vi "FPGAmain_5782_PIDtest.vi"() -> ()   [LabVIEW 2013]
uses:
  FPGA/DataMode.ctl
  FPGA/Input_5782/5782_states.ctl
  <vilib>/Platform/TimedLoop/XDataNode/timing_clust.ctl
  <vilib>/Platform/TimedLoop/XDataNode/nitl_modes.ctl
  <vilib>/Platform/TimedLoop/XDataNode/wakeup.ctl
  <vilib>/rvi/Emulation/niFpgaSctlEmulationGetInTimedLoop.vi
  <vilib>/rvi/Emulation/niFpgaEmulationReportErrorSimple.vi
  <vilib>/rvi/Emulation/niFpgaGetClockAttributes.vi
  <vilib>/rvi/eio/common/nirviEmuTemplateMethod_errors.vi
  <vilib>/rvi/Emulation/niFpgaCriticalErrorInLSC.vi
  <vilib>/rvi/FIFO/Fifo_Resource/nirvififoEmulationReadFpgaImpl.vi
  <vilib>/rvi/DataTransferAndStorage/Container/Common/niFpgaContainerGetUniqueNameForEmu.vi
  <vilib>/rvi/FIFO/Fifo_Resource/nirvififoEmulationWriteFpgaImpl.vi
  <vilib>/rvi/interface/RandomDataEmulation/nirviRandomDataFPGAFIFO.vi
  <vilib>/rvi/interface/RandomDataEmulation/niFpgaRandomDataHandleErrors.vi
  <vilib>/rvi/DataTransferAndStorage/Register/Emulation/niFpgaRegisterEmulationFpgaImpl.vi
  <instcachedir>/0/niFpgaRegisterEmulationFpgaImpl_DCF4BC0110594B98B44A971D60CEEC4D.lvgen/niFpgaRegisterEmulationFpgaImpl_DCF4BC0110594B98B44A971D60CEEC4D_003.vi
  <vilib>/Platform/TimedLoop/XDataNode/XDataNode.xnode
  <vilib>/eio/EIONode/EIONode.xnode
  <vilib>/rvi/DataTransferAndStorage/Container/XNode/niFpgaContainer.xnode
  <vilib>/rvi/FIFO/Fifo_Resource/nirvififoEmulationRead.vi
  <vilib>/rvi/FIFO/Fifo_Resource/nirvififoEmulationWrite.vi
  <vilib>/rvi/interface/RandomDataEmulation/nirviRandomDataFpgaReadWriteTemplate.vi
  <vilib>/rvi/DataTransferAndStorage/Register/Emulation/niFpgaRegisterEmulation.vi
  <vilib>/Platform/TimedLoop/XDataNode/XDNodeRunTimeDep.lvlib
panel:
  in  "Fi_delta":fxp<+/-,32,4>
  in  "Fi_start":fxp<+/-,32,4>
  in  "Kp":fxp<+/-,32,4>
  in  "Kd/Tau":fxp<+/-,32,4>
  in  "Ki*Tau":fxp<+/-,32,4>
  in  "feedback enable":bool
  in  "b_am":fxp<+/-,16,2>
  in  "a_am":fxp<+/-,16,2>
  in  "AM phase":fxp<+,64,64>
  in  "DC offset chan 0":fxp<+/-,16,16>
  in  "DC offset chan 1":fxp<+/-,16,16>
  in  "User Command Commit":bool
  in  "User Command":u8
  out "User Command Idle":bool
  out "User Command Status":u8
  in  "User Data 0":u8
  in  "User Data 1":u8
  out "PLL Locked":bool
  out "User Error":bool
  out "Configured?":bool
  in  "Continuous":bool
  in  "trigger samples":u16=1
  in  "5782 record length":u16=4000 caption="Samples Per Trigger" min=1 step=1
  in  "Trigger Acquisition":bool
  out "IO Module\\Trigger Input":bool
  in  "quiet time":u16=4000
  in  "Downsample":fxp<+,8,8>=1.0
  in  "enable filter":bool
  in  "new coeffs":bool
  in  "FIR shift":i32
  in  "FIR coeffs":fxp<+/-,18,18>[](array[numeric])
  in  "Set downsample":bool
  in  "CIC Gain":fxp<+/-,32,1>=0.00390625 format="%#_32g"
  in  "Acquisition running":bool
  in  "Phase output":fxp<+,64,64>[](array[numeric])=[0.0, 0.0, 0.0, 0.0]
  in  "Simulated phase 5782":fxp<+,64,64>[](array[numeric])=[0.0, 0.0]
  in  "Mode":T1
  in  "Phase 5782":fxp<+,64,64>[](array[numeric])=[0.0, 0.0]
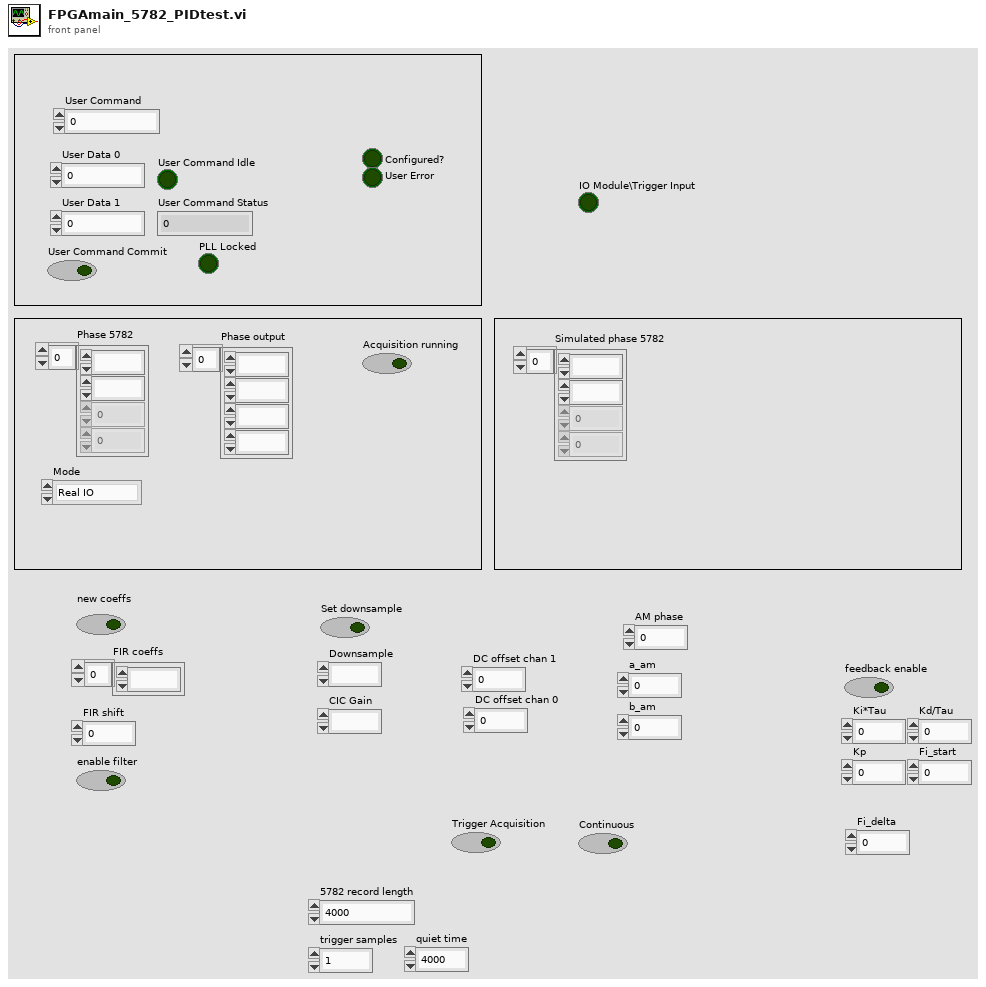
[diagram p1: front panel]
types:
  T1 = typedef "DataMode.ctl" = enum16{"Real IO", "Simulated"}
  T2 = typedef "5782_states.ctl" = enum8{"Wait for trigger", "Acquisition", "Send record length", "Quiet period"}
  T3 = typedef "XDNodeRunTimeDep.lvlib/timing_clust.ctl" = cluster{"Expected End [f-1]":u64, "Actual End [f-1]":u64, "Finished Late? [f-1]":bool, "Expected End [i-1]":u64, "Actual End [i-1]":u64, "Finished Late? [i-1]":bool, "Expected Start [i]":u64, "Actual Start [i]":u64, "Expected Start [f]":u64, "Actual Start [f]":u64, "Source Name":string, "Structure Name":string, "Period":i64, "Deadline":i64, "Offset":i64, "Start":i64, "Priority":i32, "Timeout":i32, "Mode":T4, "Wakeup Reason":T5, "Error":errorcluster, "Source Type":string, "Secondary Source Type":string, "Global End Time":u64, "Global Start Time":u64, "Frame Duration":u64, "Iteration Duration":u64, "Assigned CPU":i32, "I/O Scan Engine Mode":u32}
  T4 = typedef "XDNodeRunTimeDep.lvlib/nitl_modes.ctl" = enum32{"No Change", "Process missed periods, maintain original phase", "Discard missed periods, maintain original phase", "Process missed periods, ignore original phase", "Discard missed periods, ignore original phase"}
  T5 = typedef "XDNodeRunTimeDep.lvlib/wakeup.ctl" = enum32{"Normal", "Aborted", "Asynchronous wakeup", "Timing source error", "Timed loop error", "Timeout"}
  T6 = typedef "I16 array size 2.ctl" = i16[]
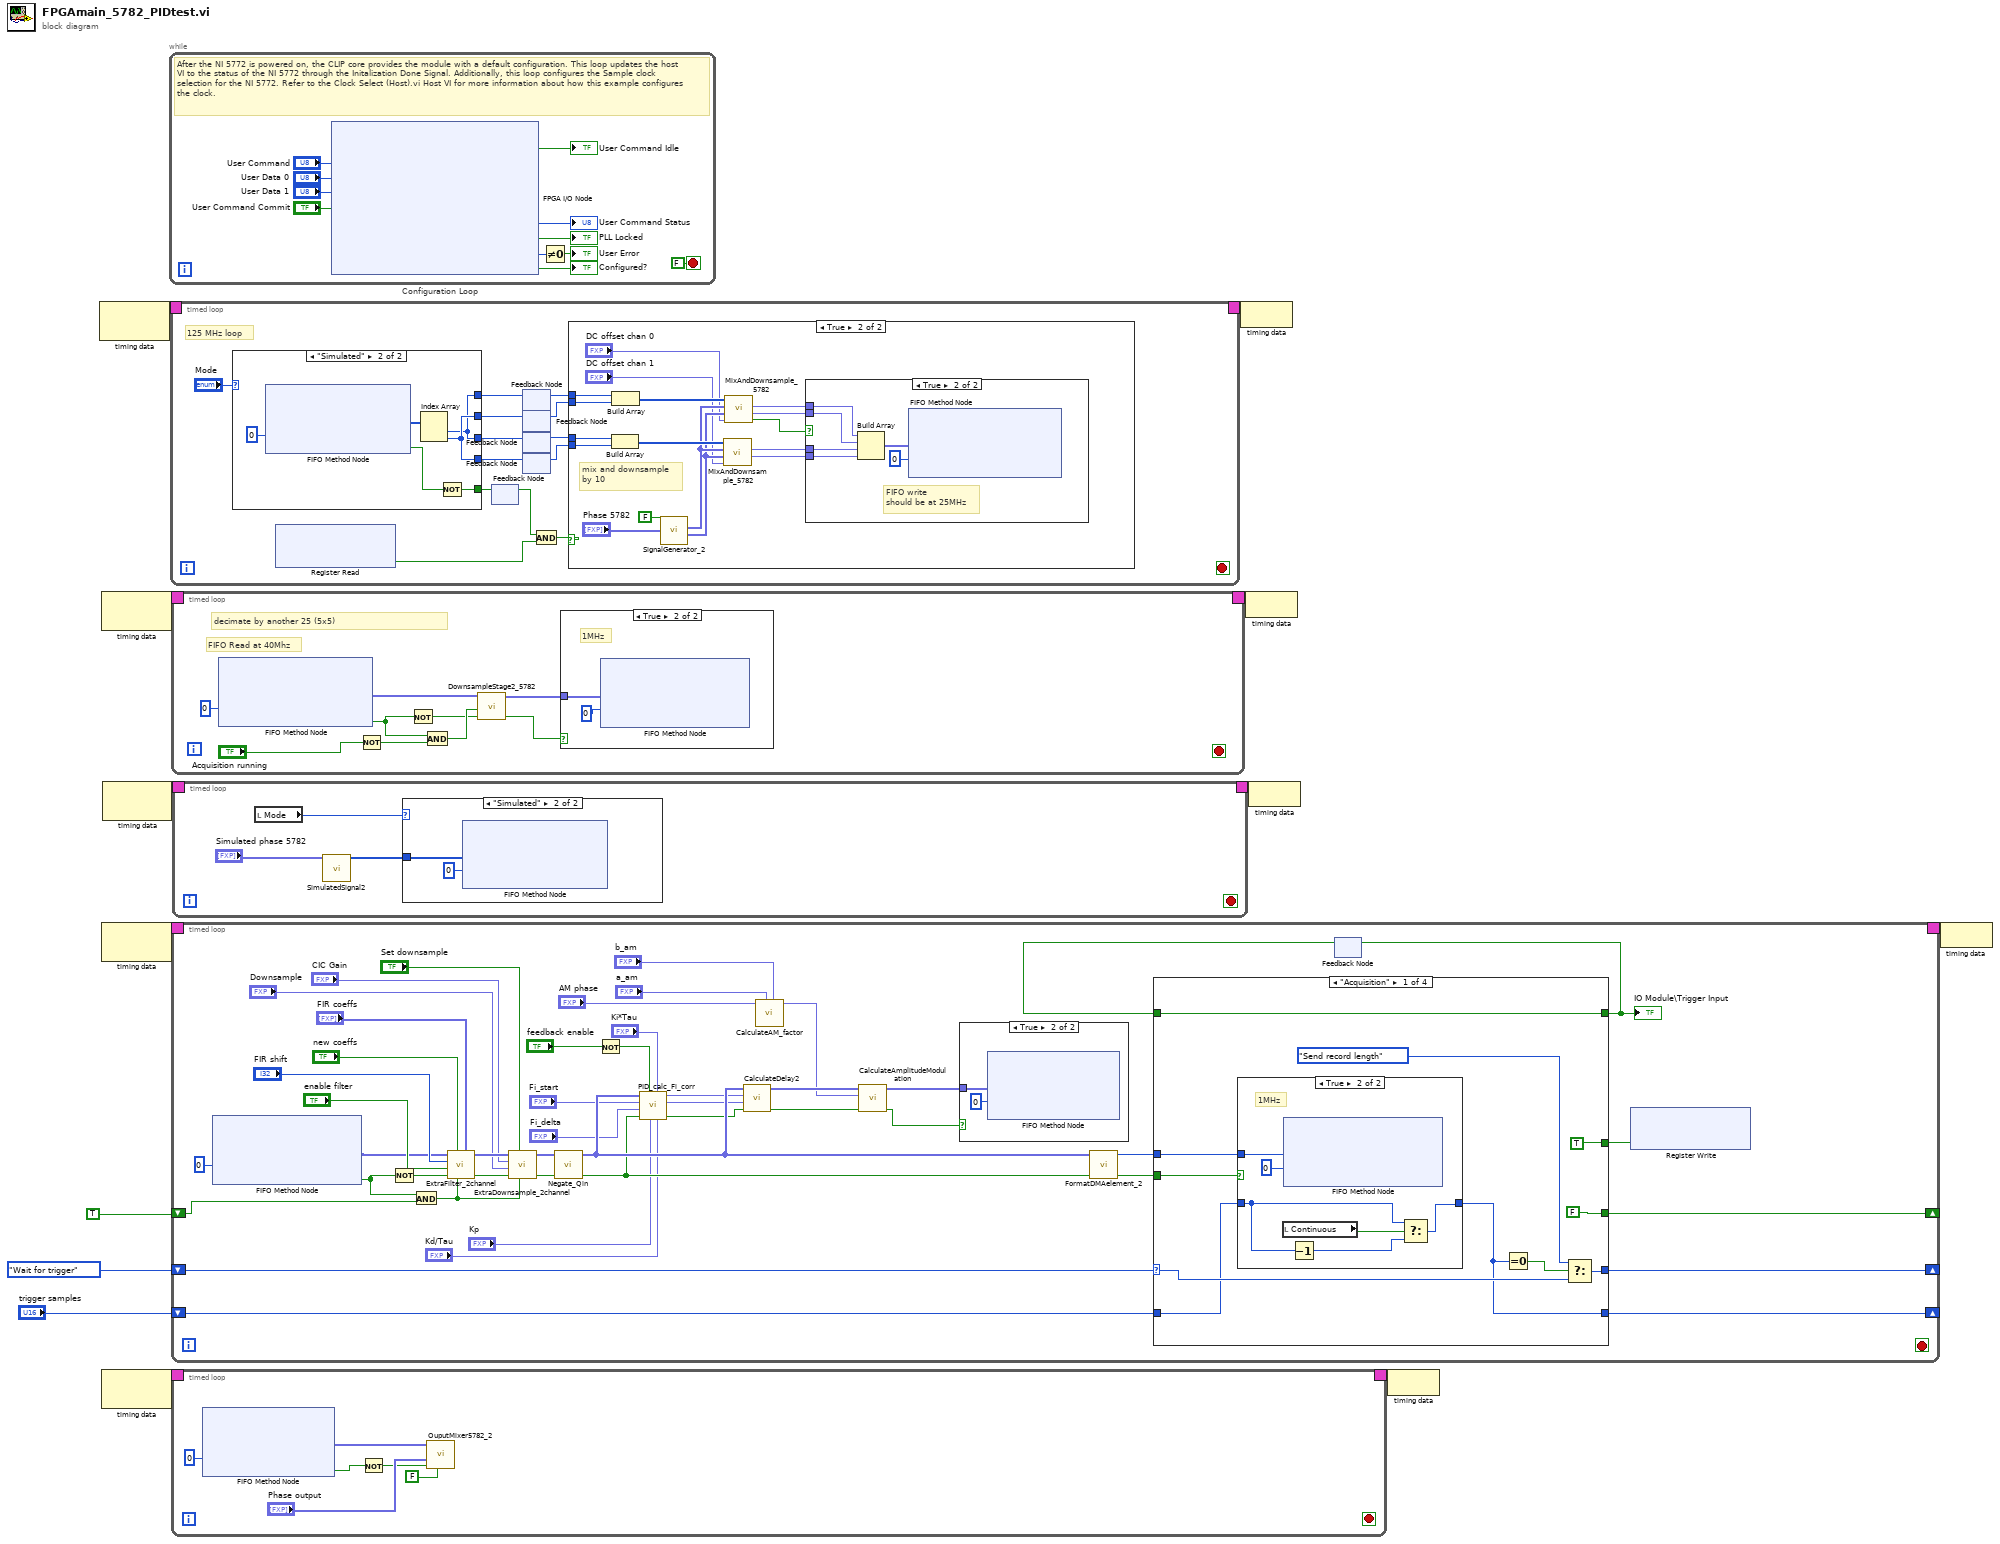
[diagram p0: block diagram]
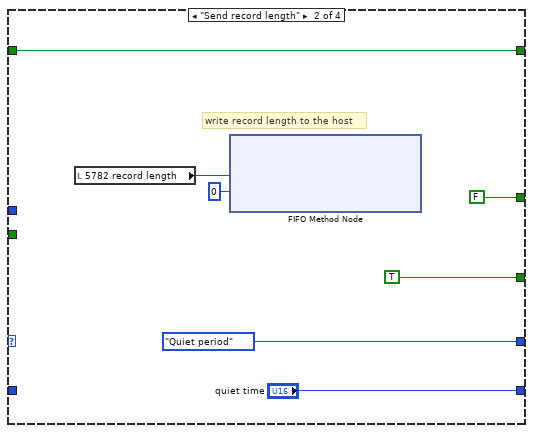
[diagram p4: hidden frame]
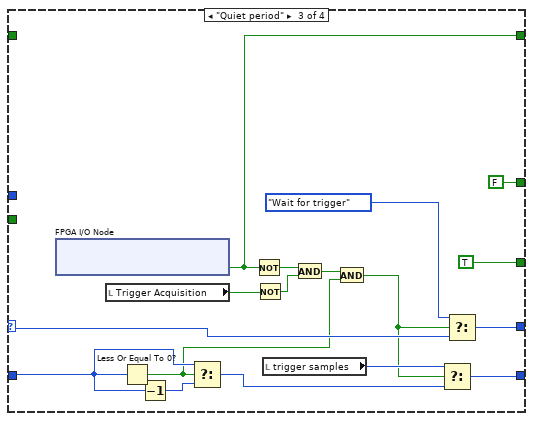
[diagram p5: hidden frame]
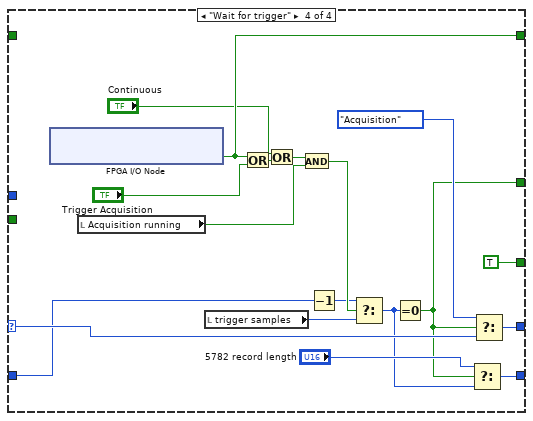
[diagram p6: hidden frame]
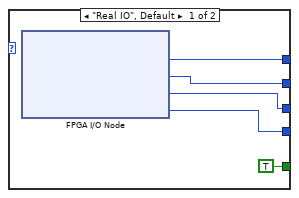
[diagram p9: hidden frame]
diagram:
  n1 = node-c288() -> (w9:T3)  [unwired: 1 in]
  n2 = node-c288() -> (w13:T3)  [unwired: 1 in]
  n3 = node-c288() -> (w7:T3)  [unwired: 1 in]
  n4 = node-c288() -> (w2:T3)  [unwired: 1 in]
  n5 = node-c288() -> (w11:T3)  [unwired: 1 in]
  n6 = while "Configuration Loop" {
    stop <- FALSE stop-if-true
    # "After the NI 5772 is powered on, the CLIP core provides the module with a default configuration. This loop updates the host VI to the status of the NI 5772 through the Initalization Done Signal. Additionally, this loop configures the Sample clock selection for the NI 5772. Refer to the Clock Select (Host).vi Host VI for more information about how this example configures the clock."
    n7 = xnode "FPGA I/O Node"("IO Module\\User Command"="User Command", "IO Module\\User Data 0"="User Data 0", "IO Module\\User Data 1"="User Data 1", "IO Module\\User Command Commit"="User Command Commit") -> ("IO Module\\User Command Idle"=→"User Command Idle":bool, "IO Module\\User Command Status"=→"User Command Status":u8, "IO Module\\PLL Locked"=→"PLL Locked":bool, "IO Module\\User Error"=w19:u8, "IO Module\\Initialization Done"=→"Configured?":bool)  [unwired: 9 in, 9 out]
    n8 = Not Equal To 0?(x=w19) -> (x != 0?=→"User Error":bool)
  }
  n9 = timed-loop {
    timing: w9 -> [_]
    timing-out: [_] -> w8
    stop <- _ stop-if-true
    # "125 MHz loop"
    n10 = case shown="\"Simulated\"" "Mode" {
      tunnel: [w65 w68] -> w35
      tunnel: [w64 w69] -> w33
      tunnel: [w63 w68] -> w31
      tunnel: [w62 w69] -> w28
      tunnel: [TRUE w66] -> w27
      frame "Real IO", Default {
        n11 = xnode "FPGA I/O Node"() -> ("IO Module\\AI 0 N-1"=w65:i16, "IO Module\\AI 0 N"=w64:i16, "IO Module\\AI 1 N-1"=w63:i16, "IO Module\\AI 1 N"=w62:i16)  [unwired: 4 in, 4 out]
      }
      frame "Simulated" {
        n12 = xnode ("FIFO Method Node")("Timeout"=0) -> ("Element"=w70:i16[], "Timed Out?"=w67:bool)  [unwired: 1 in, 1 out]
        n13 = Index Array(array=w70) -> (element #1=w68:i16, element #2=w69:i16)  [unwired: 2 in]
        n14 = Not(x=w67) -> (.not. x?=w66:bool)
      }
    }
    n15 = xnode ("Register Read")() -> ("Data"=w25:bool)  [unwired: 1 in, 1 out]
    n16 = feedback #1() -> (w26:bool)  [unwired: 1 in]
    n17 = feedback-in #1(w27) -> ()
    n18 = feedback #2() -> (w34:i16)  [unwired: 1 in]
    n19 = feedback-in #2(w35) -> ()
    n20 = feedback #3() -> (w32:i16)  [unwired: 1 in]
    n21 = feedback-in #3(w33) -> ()
    n22 = feedback #4() -> (w30:i16)  [unwired: 1 in]
    n23 = feedback-in #4(w31) -> ()
    n24 = feedback #5() -> (w29:i16)  [unwired: 1 in]
    n25 = feedback-in #5(w28) -> ()
    n26 = And(x=w26, y=w25) -> (x .and. y?=w36:bool)
    n27 = case shown="True" w36 {
      tunnel: w34 -> [_ w45]
      tunnel: w32 -> [_ w44]
      tunnel: w30 -> [_ w43]
      tunnel: w29 -> [_ w42]
      frame False {
      }
      frame True {
        # "mix and downsample\nby 10"
        n28 = Build Array(w43, w42) -> (w54:i16[])
        n29 = Build Array(w45, w44) -> (w41:i16[])
        n30 = call "SignalGenerator_2.vi"("Phase"="Phase 5782", "reset"=FALSE) -> ("Sine out"=w46:fxp<+/-,16,0>[], "Cosine out"=w47:fxp<+/-,16,0>[])  [unwired: 8 in]
        n31 = call "MixAndDownsample_5782.vi"("DC offset"="DC offset chan 1", "Sine in"=w46, "Cosine in"=w47, "Signal Input"=w54) -> ("Q out"=w49:fxp<+/-,16,14>, "I out"=w50:fxp<+/-,16,14>)  [unwired: 5 in, 1 out]
        n32 = call "MixAndDownsample_5782.vi"("DC offset"="DC offset chan 0", "Sine in"=w46, "Cosine in"=w47, "Signal Input"=w41) -> ("data valid"=w51:bool, "Q out"=w52:fxp<+/-,16,14>, "I out"=w53:fxp<+/-,16,14>)  [unwired: 5 in]
        n33 = case shown="True" w51 {
          tunnel: w52 -> [_ w60]
          tunnel: w53 -> [_ w57]
          tunnel: w50 -> [_ w56]
          tunnel: w49 -> [_ w55]
          frame False {
          }
          frame True {
            # "FIFO write\nshould be at 25MHz"
            n34 = Build Array(w57, w60, w56, w55) -> (w59:fxp<+/-,16,14>[])
            n35 = xnode ("FIFO Method Node")("Element"=w59, "Timeout"=0) -> ()  [unwired: 1 in, 2 out]
          }
        }
      }
    }
  }
  n36 = timed-loop {
    timing: w13 -> [_]
    timing-out: [_] -> w12
    stop <- _ stop-if-true
    # "FIFO Read at 40Mhz"
    # "decimate by another 25 (5x5)"
    n37 = xnode ("FIFO Method Node")("Timeout"=0) -> ("Element"=w81:fxp<+/-,16,14>[], "Timed Out?"=w77:bool)  [unwired: 1 in, 1 out]
    n38 = Not(x="Acquisition running") -> (.not. x?=w78:bool)
    n39 = Not(x=w77) -> (.not. x?=w75:bool)
    n40 = And(x=w77, y=w78) -> (x .and. y?=w76:bool)
    n41 = call "DownsampleStage2_5782.vi"("valid in"=w75, "reset"=w76, "Data in"=w81) -> ("valid out"=w79:bool, "data out"=w80:fxp<+/-,16,14>[])  [unwired: 7 in]
    n42 = case shown="True" w79 {
      tunnel: w80 -> [_ w83]
      frame False {
      }
      frame True {
        # "1MHz"
        n43 = xnode ("FIFO Method Node")("Element"=w83, "Timeout"=0) -> ()  [unwired: 1 in, 2 out]
      }
    }
  }
  n44 = timed-loop {
    timing: w7 -> [_]
    timing-out: [_] -> w6
    shift-right: [w131] -> _
    shift-left: 5782_states."Wait for trigger" ("5782 states") -> [w133]
    shift-right: [w130] -> _
    shift-left: "trigger samples" -> [w132]
    shift-right: [w112] -> _
    shift-left: TRUE -> [w115]
    stop <- _ stop-if-true
    n45 = xnode ("FIFO Method Node")("Timeout"=0) -> ("Element"=w117:fxp<+/-,16,14>[], "Timed Out?"=w116:bool)  [unwired: 1 in, 1 out]
    n46 = Not(x=w116) -> (.not. x?=w126:bool)
    n47 = And(x=w116, y=w115) -> (x .and. y?=w128:bool)
    n48 = call "ExtraFilter_2channel.vi"(5:"new coeffs"="FIR coeffs", "reset"=w128, 7:"new coeffs"="new coeffs", "valid in"=w126, "enable filter"="enable filter", "new shift"="FIR shift", "Data in"=w117) -> ("valid out"=w127:bool, "Data out"=w125:fxp<+/-,16,14>[])  [unwired: 3 in]
    n49 = call "ExtraDownsample_2channel.vi"("reset"=w128, "Set downsample"="Set downsample", "valid in"=w127, "Downsample"="Downsample", "CIC Gain"="CIC Gain", "Data in"=w125) -> ("valid out"=w107:bool, "Data out"=w108:fxp<+/-,16,14>[])  [unwired: 4 in]
    n50 = call "Negate_Qin.vi"("valid in"=w107, "Data in"=w108) -> ("valid out"=w97:bool, "Data out"=w98:fxp<+/-,16,14>[])  [unwired: 8 in]
    n51 = Not(x="feedback enable") -> (.not. x?=w92:bool)
    n52 = call "PID_calc_Fi_corr.vi"("Kd/Tau"="Kd/Tau", "Ki*Tau"="Ki*Tau", "Kp"="Kp", "Reset"=w92, "input valid"=w97, "Fi_delta"="Fi_delta", "Fi_start"="Fi_start", "Data in"=w98) -> ("output valid"=w96:bool, "cos_fi_korr"=w94:fxp<+/-,16,2>, "sin fi_korr"=w95:fxp<+/-,16,2>)  [unwired: 1 in]
    n53 = call "CalculateDelay2.vi"("input valid"=w96, "cos_fi"=w94, "sin fi"=w95, "Data in"=w98) -> ("output valid"=w105:bool, "Data out"=w106:fxp<+/-,16,14>[])  [unwired: 6 in]
    n54 = call "CalculateAM_factor.vi"("b_am"="b_am", "a_am"="a_am", "AM phase"="AM phase") -> ("AM_factor"=w99:fxp<+/-,16,2>)  [unwired: 7 in, 1 out]
    n55 = call "CalculateAmplitudeModulation.vi"("input valid"=w105, "AM_factor"=w99, "Data in"=w106) -> ("output valid"=w103:bool, "Data out"=w104:fxp<+/-,16,14>[])  [unwired: 7 in]
    n56 = case shown="True" w103 {
      tunnel: w104 -> [_ w134]
      frame False {
      }
      frame True {
        n57 = xnode ("FIFO Method Node")("Element"=w134, "Timeout"=0) -> ()  [unwired: 1 in, 2 out]
      }
    }
    n58 = call "FormatDMAelement_2.vi"("valid in"=w97, "Data in"=w98) -> ("valid out"=w113:bool, "Element1"=w114:u64)  [unwired: 8 in]
    n59 = feedback #6() -> (w110:bool)  [unwired: 1 in]
    n60 = case shown="\"Acquisition\"" w133 {
      selector: w133 -> [w146 _ w175 w195]
      tunnel: w132 -> [w142 _ w163 w182]
      tunnel: [w145 5782_states."Quiet period" ("5782 states") w174 w194] -> w131
      tunnel: [w139 "quiet time" w177 w193] -> w130
      tunnel: w114 -> [w140 _ _ _]
      tunnel: w113 -> [w141 _ _ _]
      tunnel: [FALSE TRUE TRUE TRUE] -> w112
      tunnel: [TRUE FALSE ("5782 triggered") FALSE ("5782 triggered") w186] -> w111
      tunnel: [w138 w154 w165 w185] -> w109
      tunnel: w110 -> [w138 w154 _ _]
      frame "Acquisition" {
        n61 = case shown="True" w141 {
          tunnel: w140 -> [_ w153]
          tunnel: [w147 w150] -> w139
          tunnel: w142 -> [w147 w148]
          frame False {
          }
          frame True {
            # "1MHz"
            n62 = local read "Continuous"() -> (w151:bool)
            n63 = xnode ("FIFO Method Node")("Element"=w153, "Timeout"=0) -> ()  [unwired: 1 in, 2 out]
            n64 = Decrement(x=w148) -> (x-1=w149:u16)
            n65 = Select(t=w148, s=w151, f=w149) -> (s? t:f=w150:u16)
          }
        }
        n66 = Equal To 0?(x=w139) -> (x = 0?=w143:bool)
        n67 = Select(t=5782_states."Send record length" ("5782 states"), s=w143, f=w146) -> (s? t:f=w145:T2)
      }
      frame "Send record length" {
        # "write record length to the host"
        n68 = local read "5782 record length"() -> (w156:u16)
        n69 = xnode ("FIFO Method Node")("Element"=w156, "Timeout"=0) -> ()  [unwired: 1 in, 2 out]
      }
      frame "Quiet period" {
        n70 = xnode "FPGA I/O Node"() -> ("IO Module\\Trigger Input"=w165:bool)  [unwired: 1 in, 1 out]
        n71 = local read "Trigger Acquisition"() -> (w171:bool)
        n72 = Less Or Equal To 0?(x=w163) -> (x <= 0?=w162:bool)
        n73 = Decrement(x=w163) -> (x-1=w164:u16)
        n74 = Select(t=w163, s=w162, f=w164) -> (s? t:f=w161:u16)
        n75 = Not(x=w165) -> (.not. x?=w170:bool)
        n76 = Not(x=w171) -> (.not. x?=w169:bool)
        n77 = local read "trigger samples"() -> (w176:u16)
        n78 = And(x=w170, y=w169) -> (x .and. y?=w168:bool)
        n79 = And(x=w168, y=w162) -> (x .and. y?=w173:bool)
        n80 = Select(t=w176, s=w173, f=w161) -> (s? t:f=w177:u16)
        n81 = Select(t=5782_states."Wait for trigger" ("5782 states"), s=w173, f=w175) -> (s? t:f=w174:T2)
      }
      frame "Wait for trigger" {
        n82 = xnode "FPGA I/O Node"() -> ("IO Module\\Trigger Input"=w185:bool)  [unwired: 1 in, 1 out]
        n83 = local read "Acquisition running"() -> (w187:bool)
        n84 = local read "trigger samples"() -> (w181:u16)
        n85 = Or(x=w185, y="Trigger Acquisition") -> (x .or. y?=w180:bool)
        n86 = Or(x="Continuous", y=w180) -> (x .or. y?=w178:bool)
        n87 = And(x=w178, y=w187) -> (x .and. y?=w188:bool)
        n88 = Decrement(x=w182) -> (x-1=w183:u16)
        n89 = Select(t=w183, s=w188, f=w181) -> (s? t:f=w184:u16)
        n90 = Equal To 0?(x=w184) -> (x = 0?=w186:bool)
        n91 = Select(t="5782 record length", s=w186, f=w184) -> (s? t:f=w193:u16)
        n92 = Select(t=5782_states."Acquisition" ("5782 states"), s=w186, f=w195) -> (s? t:f=w194:T2)
      }
    }
    "IO Module\\Trigger Input" <- w109
    n93 = feedback-in #6(w109) -> ()
    n94 = xnode ("Register Write")("Data"=w111) -> ()  [unwired: 1 in, 1 out]
  }
  n95 = timed-loop {
    timing: w2 -> [_]
    timing-out: [_] -> w1
    stop <- _ stop-if-true
    n96 = xnode ("FIFO Method Node")("Timeout"=0) -> ("Element"=w200:fxp<+/-,16,14>[], "Timed Out?"=w202:bool)  [unwired: 1 in, 1 out]
    n97 = Not(x=w202) -> (.not. x?=w198:bool)
    n98 = call "OuputMixer5782_2.vi"("reset"=FALSE, "valid in"=w198, "Phase output"="Phase output", "Data in"=w200) -> ()  [unwired: 7 in, 1 out]
  }
  n99 = timed-loop {
    timing: w11 -> [_]
    timing-out: [_] -> w10
    stop <- _ stop-if-true
    n100 = local read "Mode"() -> (w208:T1)
    n101 = call "SimulatedSignal2.vi"("Phase"="Simulated phase 5782") -> ("output"=w207:T6)  [unwired: 9 in, 1 out]
    n102 = case shown="\"Simulated\"" w208 {
      tunnel: w207 -> [_ w209]
      frame "Real IO", Default {
      }
      frame "Simulated" {
        n103 = xnode ("FIFO Method Node")("Element"=w209, "Timeout"=0) -> ()  [unwired: 1 in, 2 out]
      }
    }
  }
  n104 = node-c288(w8) -> ()
  n105 = node-c288(w12) -> ()
  n106 = node-c288(w10) -> ()
  n107 = node-c288(w1) -> ()
  n108 = node-c288(w6) -> ()
